vi "UpdateDeltaIndicators.vi"(6 "Lens thickness right":dbl, 10 "Lens thickness left":dbl, 11 "Target thickness":dbl) -> ()   [LabVIEW 2013]
uses:
  Global.vi
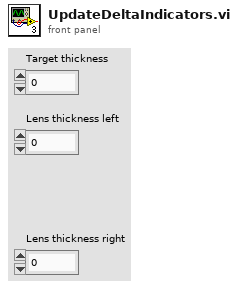
[diagram p1: front panel]
types:
  T1 = cluster{"Delta left":refnum<vi>, "Delta right":refnum<vi>, "Delta average":refnum<vi>}
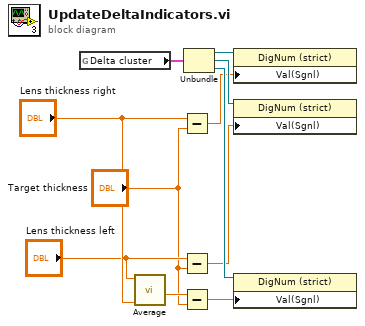
[diagram p0: block diagram]
diagram:
  n1 = global read "Global.vi" "Delta cluster"() -> (w2:T1)
  n2 = call "Average.vi"("y"="Lens thickness right", "x"="Lens thickness left") -> ("Average"=w11:dbl)  [unwired: 9 in]
  n3 = Subtract(x="Lens thickness right", y="Target thickness") -> (x-y=w4:dbl)
  n4 = Subtract(x="Lens thickness left", y="Target thickness") -> (x-y=w5:dbl)
  n5 = Subtract(x=w11, y="Target thickness") -> (x-y=w7:dbl)
  n6 = Unbundle(w2) -> ("Delta left"=w3:refnum<vi>, "Delta right"=w6:refnum<vi>, "Delta average"=w8:refnum<vi>)
  n7 = property class="DigNum (strict)"(reference=w3, "Val(Sgnl)"=w4) -> ()  [unwired: 1 in, 2 out]
  n8 = property class="DigNum (strict)"(reference=w6, "Val(Sgnl)"=w5) -> ()  [unwired: 1 in, 2 out]
  n9 = property class="DigNum (strict)"(reference=w8, "Val(Sgnl)"=w7) -> ()  [unwired: 1 in, 2 out]
